vi "Compare Headers.vi"(0 "Headers From File":string[](array[string]), 3 "Current Headers":string[](array[string]), 5 "error in (no error)":errorcluster) -> (19 "error out":errorcluster)   [LabVIEW 2015]
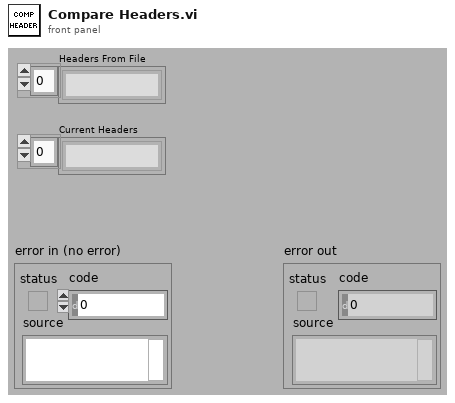
[diagram p1: front panel]
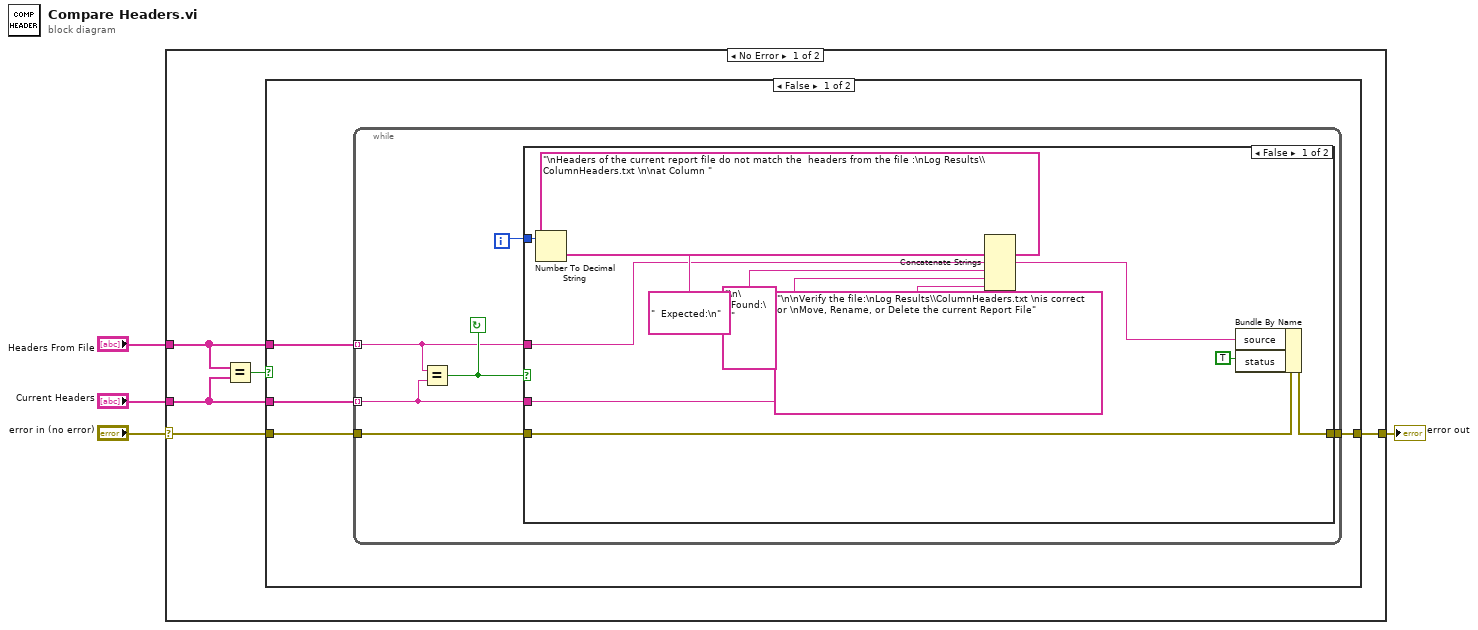
[diagram p0: block diagram]
diagram:
  n1 = case shown="No Error" "error in (no error)" {
    selector: "error in (no error)" -> [w7 w34]
    tunnel: "Headers From File" -> [w6 _]
    tunnel: "Current Headers" -> [w5 _]
    tunnel: [w8 w34] -> w2
    frame No Error {
      n2 = Equal?(x=w6, y=w5) -> (x = y?=w9:bool)
      n3 = case shown="False" w9 {
        tunnel: w7 -> [w11 w33]
        tunnel: [w10 w33] -> w8
        tunnel: w6 -> [w13 _]
        tunnel: w5 -> [w12 _]
        frame False {
          n4 = while {
            tunnel: w13 -> [w15] mode=indexing
            tunnel: w12 -> [w14] mode=indexing
            tunnel: w11 -> [w18]
            tunnel: [w17] -> w10
            i -> [w16]
            stop <- w19 continue-if-true
            n5 = Equal?(x=w15, y=w14) -> (x = y?=w19:bool)
            n6 = case shown="False" w19 {
              tunnel: w18 -> [w23 w32]
              tunnel: [w22 w32] -> w17
              tunnel: w16 -> [w31 _]
              tunnel: w15 -> [w27 _]
              tunnel: w14 -> [w25 _]
              frame False {
                n7 = Number To Decimal String(number=w31) -> (decimal integer string=w29:string)  [unwired: 1 in]
                n8 = Concatenate Strings("\nHeaders of the current report file do not match the  headers from the file :\nLog Results\\ColumnHeaders.txt \n\nat Column ", w29, "  Expected:\n" ("string"), w27, "\n\nFound:\n" ("string"), w25, "\n\nVerify the file:\nLog Results\\ColumnHeaders.txt \nis correct or \nMove, Rename, or Delete the current Report File" ("string")) -> (w21:string)
                n9 = Bundle By Name(cluster=w23, "source"=w21, "status"=TRUE) -> (w22:errorcluster)
              }
              frame True {
              }
            }
          }
        }
        frame True {
        }
      }
    }
    frame Error {
    }
  }
  "error out" <- w2
